vi "read.vi"(6 "Current Speed":refnum<vi>, 7 "Current Position":refnum<vi>, 8 "error in (no error)":errorcluster, 9 "Stop Flag Reference":refnum<vi>, 10 "VISA resource name":refnum<visa-resource-name>, 11 "QuadraturePositionDecoder in":refnum<class "QuadraturePositionDecoder.lvclass">) -> (0 "error out":errorcluster, 3 "QuadraturePositionDecoder out":refnum<class "QuadraturePositionDecoder.lvclass">)   [LabVIEW 2014, in "QuadraturePositionDecoder.lvclass"]
uses:
  QuadraturePositionDecoder.lvclass
  <vilib>/DAQmx/read.llb/DAQmx Read (Counter U32 1Chan 1Samp).vi
  <vilib>/Platform/TimedLoop/XDataNode/wakeup.ctl
  <vilib>/Platform/TimedLoop/XDataNode/XDNodeRunTimeDep.lvlib
  <vilib>/Platform/TimedLoop/XDataNode/nitl_modes.ctl
  <vilib>/Platform/TimedLoop/XDataNode/timing_clust.ctl
  <vilib>/platform/TimedLoop/XDataNode/XDataNode.xnode
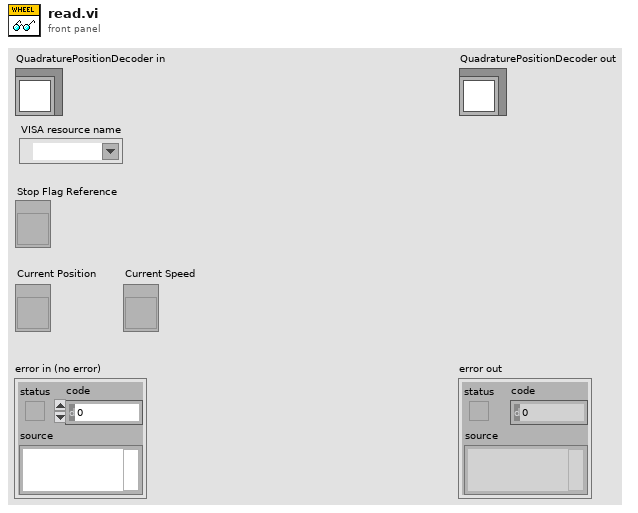
[diagram p1: front panel]
types:
  T1 = typedef "XDNodeRunTimeDep.lvlib/timing_clust.ctl" = cluster{"Expected End [f-1]":u64, "Actual End [f-1]":u64, "Finished Late? [f-1]":bool, "Expected End [i-1]":u64, "Actual End [i-1]":u64, "Finished Late? [i-1]":bool, "Expected Start [i]":u64, "Actual Start [i]":u64, "Expected Start [f]":u64, "Actual Start [f]":u64, "Source Name":string, "Structure Name":string, "Period":i64, "Deadline":i64, "Offset":i64, "Start":i64, "Priority":i32, "Timeout":i32, "Mode":T2, "Wakeup Reason":T3, "Error":errorcluster, "Source Type":string, "Secondary Source Type":string, "Global End Time":u64, "Global Start Time":u64, "Frame Duration":u64, "Iteration Duration":u64, "Assigned CPU":i32, "I/O Scan Engine Mode":u32}
  T2 = typedef "XDNodeRunTimeDep.lvlib/nitl_modes.ctl" = enum32{"No Change", "Process missed periods, maintain original phase", "Discard missed periods, maintain original phase", "Process missed periods, ignore original phase", "Discard missed periods, ignore original phase"}
  T3 = typedef "XDNodeRunTimeDep.lvlib/wakeup.ctl" = enum32{"Normal", "Aborted", "Asynchronous wakeup", "Timing source error", "Timed loop error", "Timeout"}
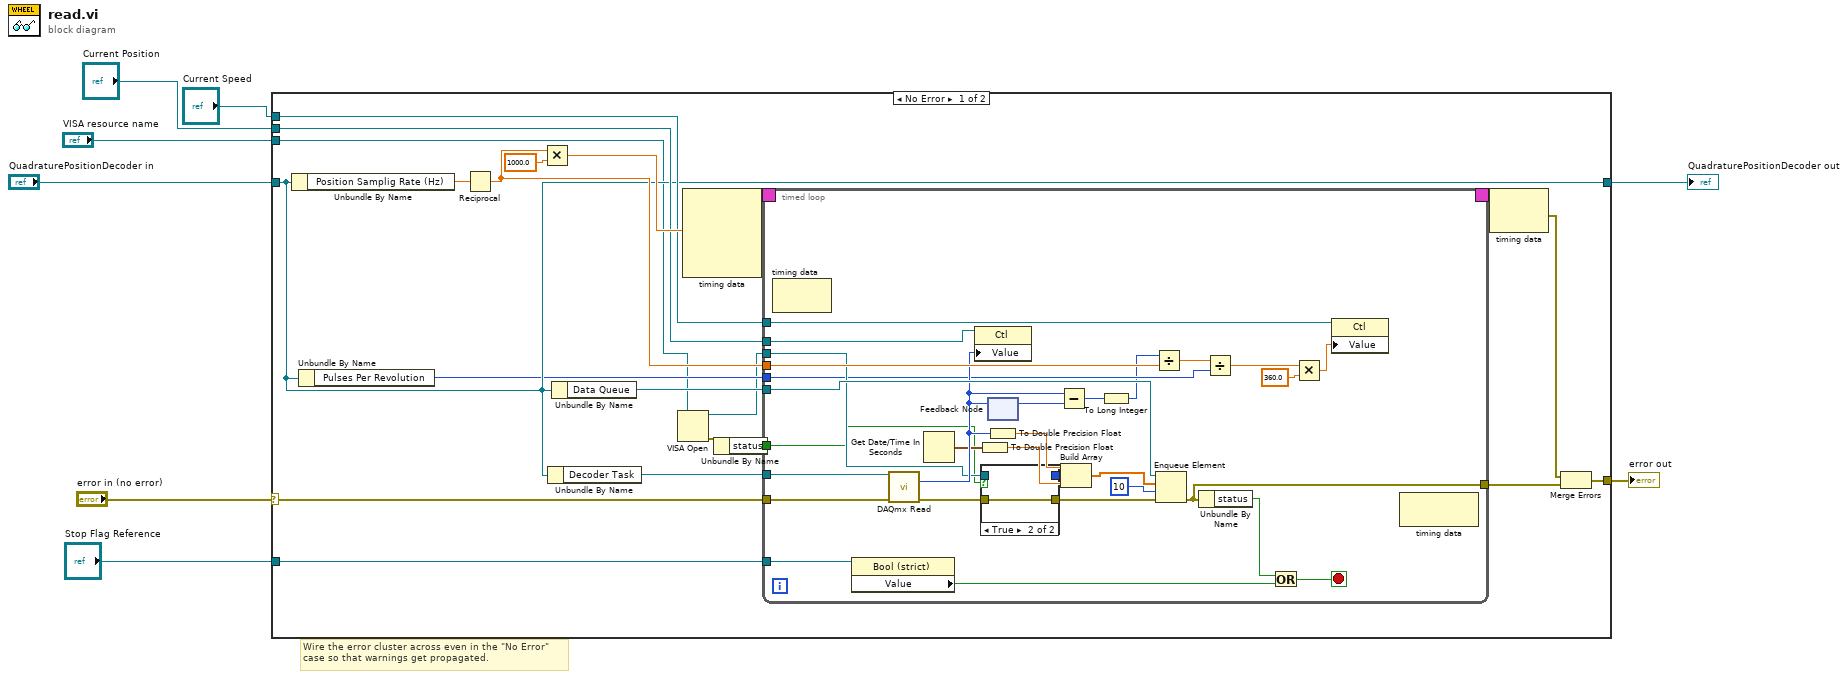
[diagram p0: block diagram]
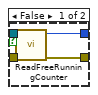
[diagram p2: hidden frame]
diagram:
  # "Wire the error cluster across even in the \"No Error\"\ncase so that warnings get propagated."
  n1 = case shown="No Error" "error in (no error)" {
    selector: "error in (no error)" -> [w27 w73]
    tunnel: [w18 w73] -> w7
    tunnel: [w14 w72] -> w5
    tunnel: "QuadraturePositionDecoder in" -> [w14 w72]
    tunnel: "VISA resource name" -> [w12 _]
    tunnel: "Stop Flag Reference" -> [w17 _]
    tunnel: "Current Speed" -> [w16 _]
    tunnel: "Current Position" -> [w15 _]
    frame No Error {
      n2 = Unbundle By Name(w14) -> ("Position Samplig Rate (Hz)"=w23:dbl)
      n3 = Unbundle By Name(w14) -> ("Pulses Per Revolution"=w13:u32)
      n4 = Reciprocal(x=w23) -> (1/x=w22:dbl)
      n5 = Multiply(x=w22, y=1000.0) -> (x*y=w21:dbl)
      n6 = Unbundle By Name(w14) -> ("Decoder Task"=w26:refnum<k21>)
      n7 = Unbundle By Name(w14) -> ("Data Queue"=w25:refnum<queue>)
      n8 = VISA Open(VISA resource name=w12) -> (VISA resource name=w11:refnum<visa-resource-name>, error out=w10:errorcluster)  [unwired: 4 in]
      n9 = node-c288(w21) -> (w29:T1)  [unwired: 3 in]
      n10 = Unbundle By Name(w10) -> ("status"=w9:bool)
      n11 = timed-loop {
        tunnel: w26 -> [w59]
        tunnel: w27 -> [w58]
        tunnel: [w49] -> w20
        tunnel: w25 -> [w53]
        timing: w29 -> [_]
        timing-out: [_] -> w28
        tunnel: w11 -> [w43]
        tunnel: w22 -> [w50]
        tunnel: w17 -> [w48]
        tunnel: w16 -> [w46]
        tunnel: w15 -> [w45]
        tunnel: w13 -> [w36]
        tunnel: w9 -> [w30]
        stop <- w57 stop-if-true
        n12 = node-c288() -> ()  [unwired: 1 in, 1 out]
        n13 = property class="Bool (strict)"(reference=w48) -> ("Value"=w47:bool)  [unwired: 1 in, 2 out]
        n14 = call-poly <vilib>:"DAQmx Read.vi"("task/channels in"=w59, "error in"=w58) -> ("data"=w44:u32, "error out"=w42:errorcluster)  [unwired: 11 in, 1 out]
        n15 = Get Date/Time In Seconds() -> (seconds since 1Jan1904=w39:timestamp)
        n16 = property class="Ctl"(reference=w45, "Value"=w44) -> ()  [unwired: 1 in, 2 out]
        n17 = To Double Precision Float(number=w39) -> (double precision float=w38:dbl)
        n18 = case shown="True" w30 {
          tunnel: w43 -> [w63 _]
          tunnel: w42 -> [w62 w64]
          tunnel: [w61 w64] -> w41
          tunnel: [w60 _] -> w40
          frame False {
            n19 = call "ReadFreeRunningCounter.vi"("error in"=w62, "VISA resource name"=w63) -> ("error out"=w61:errorcluster, "Counter Data"=w60:u32)  [unwired: 8 in]
          }
          frame True {
          }
        }
        n20 = feedback-in #1(w44) -> ()
        n21 = feedback #1() -> (w52:u32)  [unwired: 1 in]
        n22 = To Double Precision Float(number=w44) -> (double precision float=w51:dbl)
        n23 = Subtract(x=w44, y=w52) -> (x-y=w35:u32)
        n24 = Build Array(w51, w40, w38) -> (w54:dbl[])
        n25 = To Long Integer(number=w35) -> (32bit integer=w34:i32)
        n26 = Divide(x=w34, y=w50) -> (x/y=w37:dbl)
        n27 = Enqueue Element(queue=w53, element=w54, timeout in ms (-1)=10, error in (no error)=w41) -> (error out=w49:errorcluster)  [unwired: 2 out]
        n28 = Unbundle By Name(w49) -> ("status"=w56:bool)
        n29 = Divide(x=w37, y=w36) -> (x/y=w33:dbl)
        n30 = Or(x=w56, y=w47) -> (x .or. y?=w57:bool)
        n31 = Multiply(x=w33, y=360.0) -> (x*y=w32:dbl)
        n32 = property class="Ctl"(reference=w46, "Value"=w32) -> ()  [unwired: 1 in, 2 out]
        n33 = node-c288() -> ()  [unwired: 1 in, 1 out]
      }
      n34 = node-c288(w28) -> (w19:errorcluster)
      n35 = Merge Errors(w19, w20) -> (w18:errorcluster)
    }
    frame Error {
    }
  }
  "error out" <- w7
  "QuadraturePositionDecoder out" <- w5
